vi "mbed PID Hello World.vi"() -> ()   [LabVIEW 2009]
uses:
  <vilib>/Platform/TimedLoop/XDataNode/XDataNode.xnode
  <vilib>/Platform/TimedLoop/XDataNode/loadlvalarms.vi
  <vilib>/Platform/TimedLoop/XDataNode/timing_clust.ctl
  <vilib>/Platform/TimedLoop/XDataNode/nitl_modes.ctl
  <vilib>/Platform/TimedLoop/XDataNode/wakeup.ctl
  <vilib>/Platform/TimedLoop/XDataNode/XDNodeRunTimeDep.lvlib
panel:
  in  "Serial Port":refnum<visa-resource-name>
  in  "DC Offset":dbl=50.0 min=0.0
  out "Process Variable from mbed":dbl
  out "Output To mbed":dbl
  in  "Integral Enabled":bool=TRUE
  in  "Kd":dbl
  in  "Ki":dbl
  in  "Kp":dbl
  out "Setpoint and Process Variable":dynamicdata(graph)
  in  "stop":bool
  out "Error":dbl
  in  "Setpoint":dbl(slide) step=1.18471116e-315 scale=0.0..100.0
  # "The Plant - mbed"
  # "The Controller"
  # "+"
  # "-"
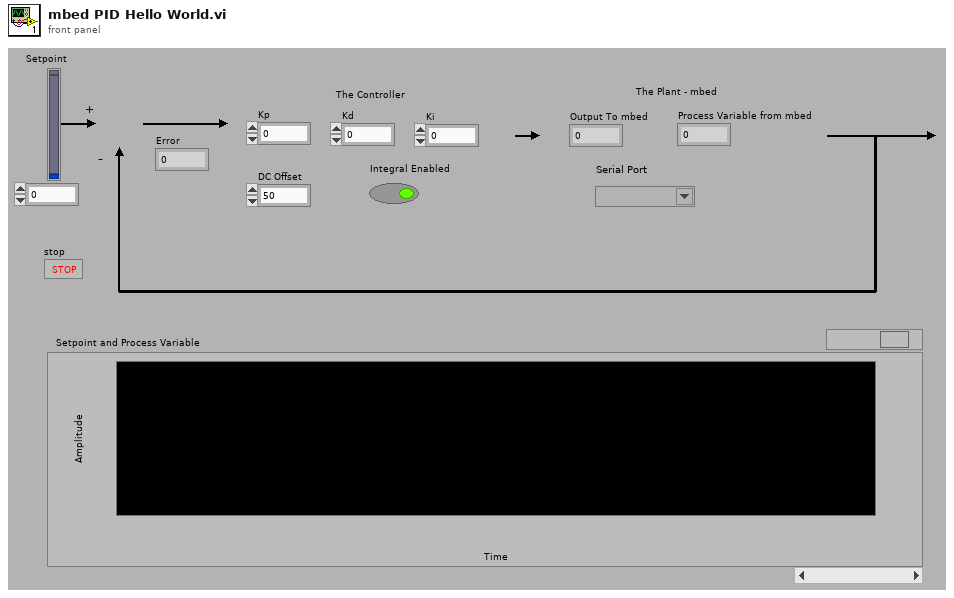
[diagram p1: front panel]
types:
  T1 = typedef "XDNodeRunTimeDep.lvlib/timing_clust.ctl" = cluster{"Expected End [f-1]":u64, "Actual End [f-1]":u64, "Finished Late? [f-1]":bool, "Expected End [i-1]":u64, "Actual End [i-1]":u64, "Finished Late? [i-1]":bool, "Expected Start [i]":u64, "Actual Start [i]":u64, "Expected Start [f]":u64, "Actual Start [f]":u64, "Source Name":string, "Structure Name":string, "Period":i64, "Deadline":i64, "Offset":i64, "Start":i64, "Priority":i32, "Timeout":i32, "Mode":T2, "Wakeup Reason":T3, "Error":errorcluster, "Source Type":string, "Secondary Source Type":string, "Global End Time":u64, "Global Start Time":u64, "Frame Duration":u64, "Iteration Duration":u64, "Assigned CPU":i32, "I/O Scan Engine Mode":u32}
  T2 = typedef "XDNodeRunTimeDep.lvlib/nitl_modes.ctl" = enum32{"No Change", "Process missed periods, maintain original phase", "Discard missed periods, maintain original phase", "Process missed periods, ignore original phase", "Discard missed periods, ignore original phase"}
  T3 = typedef "XDNodeRunTimeDep.lvlib/wakeup.ctl" = enum32{"Normal", "Aborted", "Asynchronous wakeup", "Timing source error", "Timed loop error", "Timeout"}
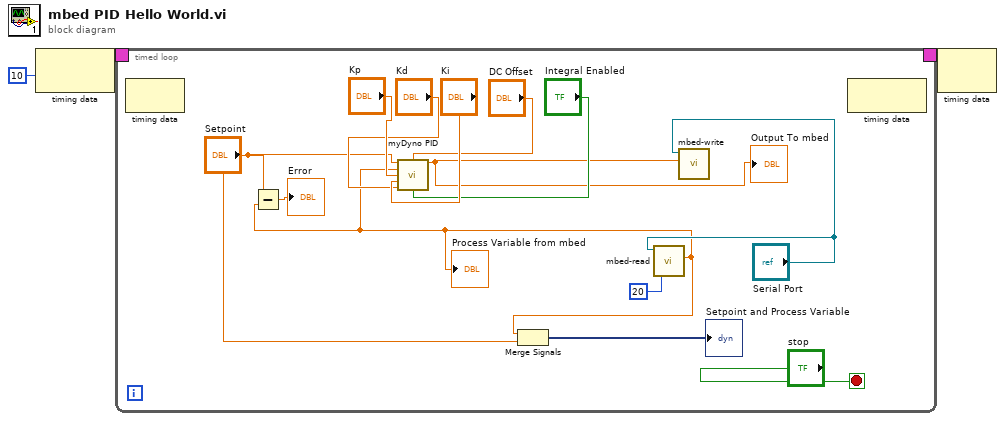
[diagram p0: block diagram]
diagram:
  n1 = node-c288(i64 10 ("Period")) -> (w3:T1)
  n2 = timed-loop {
    timing: w3 -> [_]
    timing-out: [_] -> w2
    stop <- "stop" stop-if-true
    n3 = node-c288() -> ()  [unwired: 1 in, 1 out]
    n4 = call "mbed-read.vi"("timeout (10sec)"=u32 20, "Serial Port"="Serial Port") -> ("Number"=w5:dbl)  [unwired: 2 in, 3 out]
    "Process Variable from mbed" <- w5
    n5 = Subtract(x="Setpoint", y=w5) -> (x-y=→"Error":dbl)
    n6 = call "myDyno PID.vi"("Setpoint"="Setpoint", "DC Offset"="DC Offset", "Process Variable"=w5, "Kp"="Kp", "Ki"="Ki", "Kd"="Kd", "Integral Enabled"="Integral Enabled") -> ("Control Signal (% Duty)"=w4:dbl)  [unwired: 7 in, 1 out]
    "Output To mbed" <- w4
    n7 = Merge Signals(w5, "Setpoint") -> (→"Setpoint and Process Variable":dynamicdata)
    n8 = call "mbed-write.vi"("Serial Port"="Serial Port", "Number"=w4) -> ()  [unwired: 5 in, 1 out]
    n9 = node-c288() -> ()  [unwired: 1 in, 1 out]
  }
  n10 = node-c288(w2) -> ()  [unwired: 1 out]
